vi "FL Set Rule.vi"(4 "consequent implication":T1 items=["Minimum", "Product"], 5 "antecedent connective":T2 items=["AND (Minimum)", "AND (Product)", "OR (Maximum)", "OR (Probabilistic)"], 6 "consequents":T3[](array[typedef]) {"Var Index" min=0; "Cond" items=["=", "!="]; "MF Index" min=0}, 7 "antecedents":T5[](array[typedef]) {"Var Index" min=0; "Cond" items=["=", "!="]; "MF Index" min=0}, 8 "error in (no error)":errorcluster, 9 "degree of support (1)":dbl=1.0, 10 "rule index":i32, 11 "fuzzy system in":T6 {"user MF interpolating polynomials"."coa_x(y) coeff" format="%.4g"; "user MF interpolating polynomials"."Area(y) coeff" format="%.4g"; "user MF interpolating polynomials"."X(y) coeff" format="%.4g"; "user MF interpolating polynomials"."Y(x) coeff" format="%.4g"; "user MF interpolating polynomials"."Y" format="%.4g"; "user MF interpolating polynomials"."X" format="%.4g"; "defuzzification method" items=["Center of Area", "Modified Center of Area", "Center of Sums", "Center of Maximum", "Mean of Maximum"]; "rules"."consequents"."Var Index" min=0; "rules"."consequents"."Cond" items=["=", "!="]; "rules"."consequents"."MF Index" min=0; "rules"."antecedents"."Var Index" min=0; "rules"."antecedents"."Cond" items=["=", "!="]; "rules"."antecedents"."MF Index" min=0; "rules"."consequent implication" items=["Minimum", "Product"]; "rules"."antecedent connective" items=["AND (Minimum)", "AND (Product)", "OR (Maximum)", "OR (Probabilistic)"]; "output variables"."MFs"."shape" items=["Triangle", "Trapezoid", "Singleton", "Sigmoid", "Gaussian", "User-Defined"]; "input variables"."MFs"."shape" items=["Triangle", "Trapezoid", "Singleton", "Sigmoid", "Gaussian", "User-Defined"]}) -> (0 "error out":errorcluster, 3 "fuzzy system out":T6 {"user MF interpolating polynomials"."coa_x(y) coeff" format="%.4g"; "user MF interpolating polynomials"."Area(y) coeff" format="%.4g"; "user MF interpolating polynomials"."X(y) coeff" format="%.4g"; "user MF interpolating polynomials"."Y(x) coeff" format="%.4g"; "user MF interpolating polynomials"."Y" format="%.4g"; "user MF interpolating polynomials"."X" format="%.4g"; "defuzzification method" items=["Center of Area", "Modified Center of Area", "Center of Sums", "Center of Maximum", "Mean of Maximum"]; "rules"."consequents"."Var Index" min=0; "rules"."consequents"."Cond" items=["=", "!="]; "rules"."consequents"."MF Index" min=0; "rules"."antecedents"."Var Index" min=0; "rules"."antecedents"."Cond" items=["=", "!="]; "rules"."antecedents"."MF Index" min=0; "rules"."consequent implication" items=["Minimum", "Product"]; "rules"."antecedent connective" items=["AND (Minimum)", "AND (Product)", "OR (Maximum)", "OR (Probabilistic)"]; "output variables"."MFs"."shape" items=["Triangle", "Trapezoid", "Singleton", "Sigmoid", "Gaussian", "User-Defined"]; "input variables"."MFs"."shape" items=["Triangle", "Trapezoid", "Singleton", "Sigmoid", "Gaussian", "User-Defined"]})   [LabVIEW 2020, in "NI_Fuzzy_Logic_API.lvlib"]
doc: "Modifies the antecedents, consequents, or relationships of a rule in a fuzzy system."
uses:
  <vilib>/addons/Fuzzy Logic/NI_Fuzzy_Logic_API.lvlib
  <vilib>/addons/Fuzzy Logic/TypeDefs/FL System.ctl
  <vilib>/addons/Fuzzy Logic/TypeDefs/FL Variable.ctl
  <vilib>/addons/Fuzzy Logic/TypeDefs/FL Membership Function.ctl
  <vilib>/addons/Fuzzy Logic/TypeDefs/FL Membership Function Shape.ctl
  <vilib>/addons/Fuzzy Logic/TypeDefs/FL Rule.ctl
  <vilib>/addons/Fuzzy Logic/TypeDefs/FL Antecedent.ctl
  <vilib>/addons/Fuzzy Logic/TypeDefs/FL Modifier.ctl
  <vilib>/addons/Fuzzy Logic/TypeDefs/FL Antecedent Connective.ctl
  <vilib>/addons/Fuzzy Logic/TypeDefs/FL Consequent.ctl
  <vilib>/addons/Fuzzy Logic/TypeDefs/FL Consequent Implication.ctl
  <vilib>/addons/Fuzzy Logic/TypeDefs/FL Defuzzification.ctl
  <vilib>/addons/Fuzzy Logic/TypeDefs/FL Interpolating polynomials.ctl
panel:
  # "IF"
  # "THEN"
  # "IF"
  # "THEN"
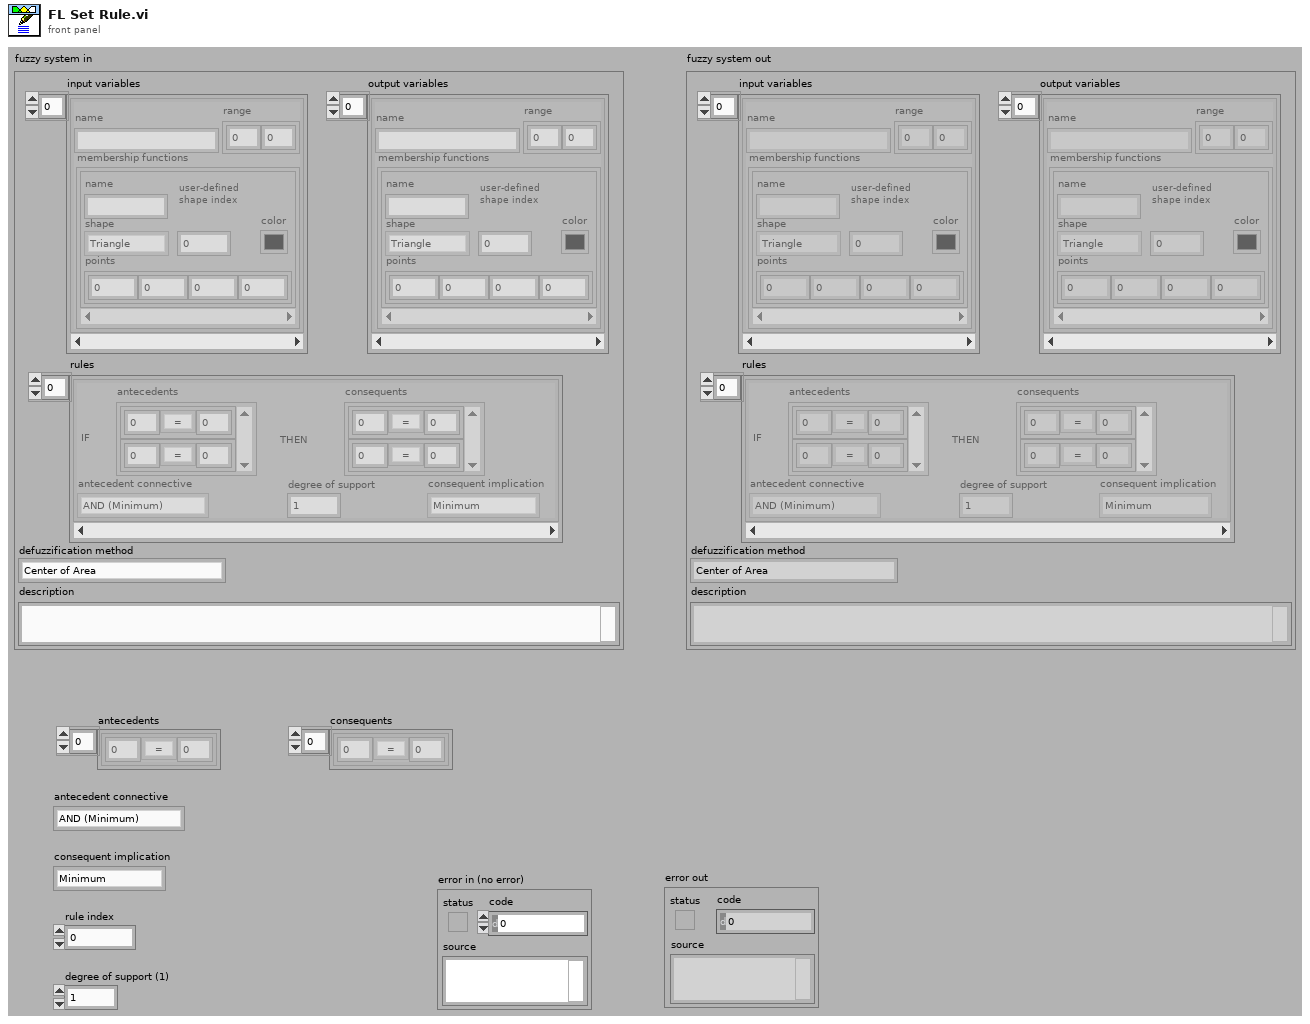
[diagram p1: front panel]
types:
  T1 = typedef "NI_Fuzzy_Logic_API.lvlib/FL Consequent Implication.ctl" = u16
  T2 = typedef "NI_Fuzzy_Logic_API.lvlib/FL Antecedent Connective.ctl" = u16
  T3 = typedef "NI_Fuzzy_Logic_API.lvlib/FL Consequent.ctl" = cluster{"Var Index":i32, "MF Index":i32, "Cond":T4}
  T4 = typedef "NI_Fuzzy_Logic_API.lvlib/FL Modifier.ctl" = u16
  T5 = typedef "NI_Fuzzy_Logic_API.lvlib/FL Antecedent.ctl" = cluster{"Var Index":i32, "MF Index":i32, "Cond":T4}
  T6 = typedef "NI_Fuzzy_Logic_API.lvlib/FL System.ctl" = cluster{"input variables":T7[], "output variables":T7[], "rules":T10[], "defuzzification method":T11, "description":string, "user MF interpolating polynomials":T12[]}
  T7 = typedef "NI_Fuzzy_Logic_API.lvlib/FL Variable.ctl" = cluster{"name":string, "range":dbl[], "MFs":T8[]}
  T8 = typedef "NI_Fuzzy_Logic_API.lvlib/FL Membership Function.ctl" = cluster{"name":string, "shape":T9, "points":dbl[], "color":u32, "user-defined shape index":i32}
  T9 = typedef "NI_Fuzzy_Logic_API.lvlib/FL Membership Function Shape.ctl" = u16
  T10 = typedef "NI_Fuzzy_Logic_API.lvlib/FL Rule.ctl" = cluster{"antecedents":T5[], "antecedent connective":T2, "consequents":T3[], "consequent implication":T1, "degree of support":dbl}
  T11 = typedef "NI_Fuzzy_Logic_API.lvlib/FL Defuzzification.ctl" = u16
  T12 = typedef "NI_Fuzzy_Logic_API.lvlib/FL Interpolating polynomials.ctl" = cluster{"X":dbl[], "Y":dbl[], "Y(x) coeff":dbl[][], "X(y) coeff":dbl[][], "Area(y) coeff":dbl[][], "coa_x(y) coeff":dbl[][]}
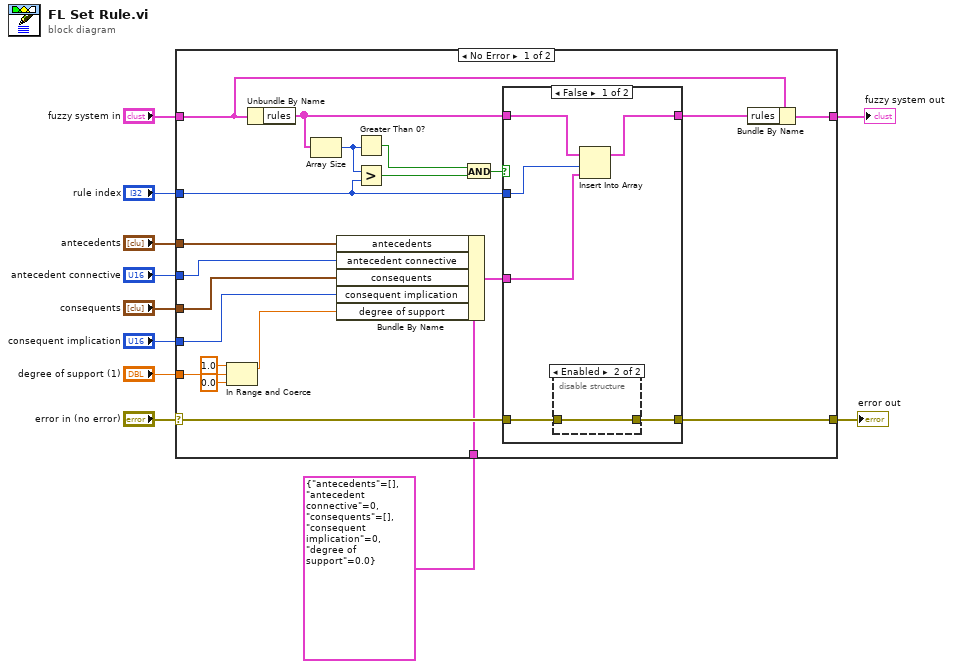
[diagram p0: block diagram]
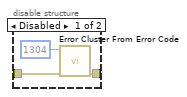
[diagram p2: hidden frame]
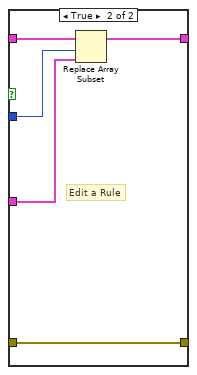
[diagram p3: hidden frame]
diagram:
  n1 = case shown="No Error" "error in (no error)" {
    selector: "error in (no error)" -> [w19 w48]
    tunnel: "fuzzy system in" -> [w32 w49]
    tunnel: [w31 w49] -> w10
    tunnel: "rule index" -> [w27 _]
    tunnel: "antecedents" -> [w17 _]
    tunnel: "antecedent connective" -> [w16 _]
    tunnel: "consequents" -> [w15 _]
    tunnel: "degree of support (1)" -> [w21 _]
    tunnel: "consequent implication" -> [w14 _]
    tunnel: [w20 w48] -> w2
    tunnel: T10 {"antecedents"=[], "antecedent connective"=0, "consequents"=[], "consequent implication"=0, "degree of support"=0.0} ("element") -> [w18 _]
    frame No Error {
      n2 = In Range and Coerce(upper limit=1.0, x=w21, lower limit=0.0) -> (coerced(x)=w13:dbl)  [unwired: 1 out]
      n3 = Unbundle By Name(w32) -> ("rules"=w29:T10[])
      n4 = Array Size(array=w29) -> (size(s)=w26:i32)
      n5 = Bundle By Name(cluster=w18, "antecedents"=w17, "antecedent connective"=w16, "consequents"=w15, "consequent implication"=w14, "degree of support"=w13) -> (w12:T10)
      n6 = Greater Than 0?(x=w26) -> (x > 0?=w25:bool)
      n7 = Greater?(x=w26, y=w27) -> (0:w28:bool)
      n8 = And(x=w25, y=w28) -> (x .and. y?=w24:bool)
      n9 = case shown="False" w24 {
        tunnel: w27 -> [w34 w47]
        tunnel: w12 -> [w35 w46]
        tunnel: [w36 w45] -> w30
        tunnel: w29 -> [w33 w44]
        tunnel: [w37 w43] -> w20
        tunnel: w19 -> [w38 w43]
        frame False {
          n10 = disable-structure shown="Enabled" {
            disable-tunnel: w38 -> [w41 w42]
            disable-tunnel: [w40 w42] -> w37
            frame Disabled {
              n11 = call <vilib>:"Error Cluster From Error Code.vi"("error in (no error)"=w41, "error code (0)"=1304) -> ("error out"=w40:errorcluster)  [unwired: 1 in, 6 out]
            }
            frame Enabled {
            }
          }
          n12 = Insert Into Array(array=w33, index=w34, new element=w35) -> (w36:T10[])
        }
        frame True {
          # "Edit a Rule"
          n13 = Replace Array Subset(array=w44, new element=w46, index=w47) -> (w45:T10[])
        }
      }
      n14 = Bundle By Name(cluster=w32, "rules"=w30) -> (w31:T6)
    }
    frame Error {
    }
  }
  "fuzzy system out" <- w10
  "error out" <- w2
